vi "DtaNmDispOpt.vi"(8 "error in (no error)":errorcluster caption="entrée d'erreur (pas d'erreur)", 11 "BaseDevice en entrée":refnum<class "BaseDevice.lvclass"> caption="DNL_LabVIEW Object in") -> (0 "error out":errorcluster caption="sortie d'erreur", 1 "ArrDisplayNames":string[](array[string]), 2 "DisplayNames":string[](array[string]), 3 "BaseDevice en sortie":refnum<class "BaseDevice.lvclass"> caption="DNL_LabVIEW Object out")   [LabVIEW 2019, in "BaseDevice.lvclass"]
uses:
  BaseDevice.lvclass
  BaseDevice.lvclass/BaseDevice.ctl
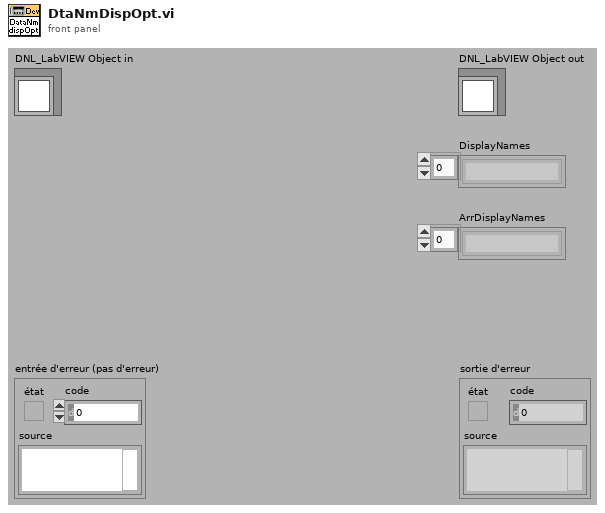
[diagram p1: front panel]
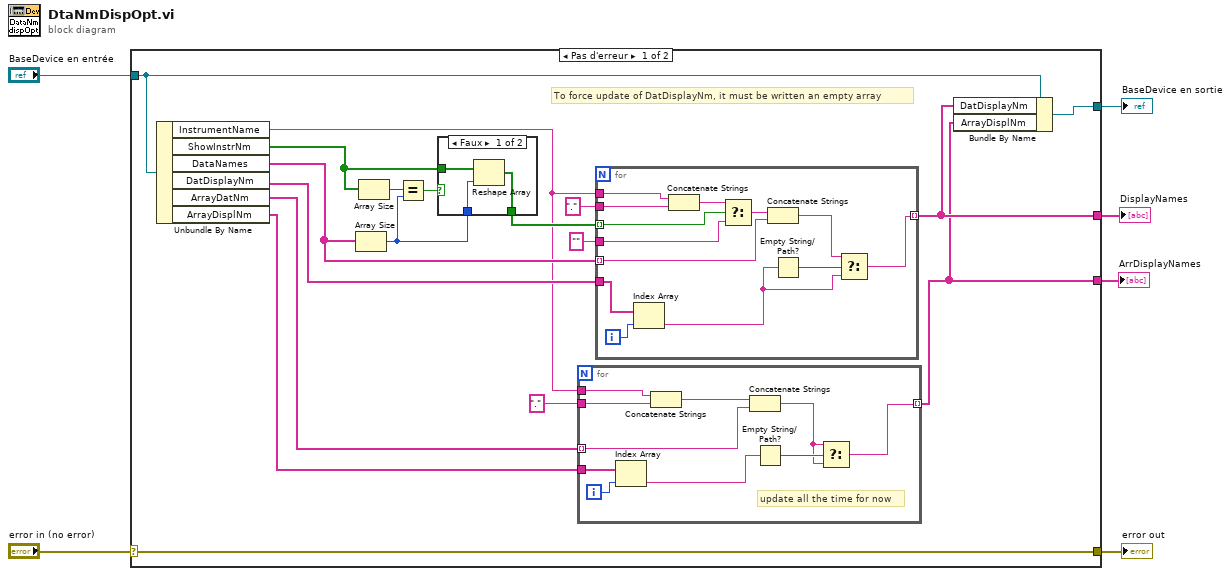
[diagram p0: block diagram]
diagram:
  n1 = case shown="Pas d'erreur" "error in (no error)" {
    selector: "error in (no error)" -> [w24 w53]
    tunnel: [w24 w53] -> w5
    tunnel: [w20 w52] -> w3
    tunnel: "BaseDevice en entrée" -> [w21 w52]
    tunnel: [w19 _] -> w2
    tunnel: [w7 _] -> w1
    frame No Error {
      # "To force update of DatDisplayNm, it must be written an empty array"
      n2 = Unbundle By Name(w21) -> ("InstrumentName"=w11:string, "ShowInstrNm"=w14:bool[], "DataNames"=w17:string[], "DatDisplayNm"=w18:string[], "ArrayDatNm"=w9:string[], "ArrayDisplNm"=w8:string[])
      n3 = Array Size(array=w17) -> (size(s)=w13:i32)
      n4 = Array Size(array=w14) -> (size(s)=w16:i32)
      n5 = Equal?(x=w16, y=w13) -> (x = y?=w15:bool)
      n6 = case shown="Faux" w15 {
        tunnel: w14 -> [w37 w38]
        tunnel: w13 -> [w36 _]
        tunnel: [w35 w38] -> w12
        frame False {
          n7 = Reshape Array(w37, w36) -> (w35:bool[])
        }
        frame True {
        }
      }
      n8 = for {
        tunnel: w9 -> [w28] mode=indexing
        tunnel: w11 -> [w34]
        tunnel: "." ("chaîne") -> [w33]
        tunnel: [w27] -> w7 mode=indexing
        tunnel: w8 -> [w31]
        i -> [w30]
        # "update all the time for now"
        n9 = Index Array(array=w31, index=w30) -> (element=w29:string)
        n10 = Concatenate Strings(w34, w33) -> (w26:string)
        n11 = Concatenate Strings(w26, w28) -> (w25:string)
        n12 = Empty String/Path?(string/path=w29) -> (empty?=w32:bool)
        n13 = Select(t=w25, s=w32, f=w25) -> (s? t:f=w27:string)
      }
      n14 = for {
        tunnel: w17 -> [w41] mode=indexing
        tunnel: w11 -> [w51]
        tunnel: "." ("chaîne") -> [w50]
        tunnel: [w39] -> w19 mode=indexing
        tunnel: "" ("cas faux") -> [w48]
        tunnel: w18 -> [w44]
        tunnel: w12 -> [w45] mode=indexing
        i -> [w43]
        n15 = Index Array(array=w44, index=w43) -> (element=w42:string)
        n16 = Concatenate Strings(w51, w50) -> (w49:string)
        n17 = Select(t=w49, s=w45, f=w48) -> (s? t:f=w47:string)
        n18 = Concatenate Strings(w47, w41) -> (w40:string)
        n19 = Empty String/Path?(string/path=w42) -> (empty?=w46:bool)
        n20 = Select(t=w40, s=w46, f=w42) -> (s? t:f=w39:string)
      }
      n21 = Bundle By Name(cluster=w21, "DatDisplayNm"=w19, "ArrayDisplNm"=w7) -> (w20:refnum<class "BaseDevice.lvclass">)
    }
    frame Error {
    }
  }
  "error out" <- w5
  "BaseDevice en sortie" <- w3
  "DisplayNames" <- w2
  "ArrDisplayNames" <- w1
